vi "Create.vi"(5 "FlexLogger_gRPC in":refnum<class "FlexLogger_gRPC.lvclass">, 8 "error in (no error)":errorcluster, 10 "PortID [Autodetect]":u16, 11 "Address":string="127.0.0.1") -> (0 "error out":errorcluster, 3 "FlexLogger_gRPC out":refnum<class "FlexLogger_gRPC.lvclass">)   [LabVIEW 2020, in "FlexLogger_gRPC.lvlib" / "FlexLogger_gRPC.lvclass"]
doc: "Constructor for the grpc object."
uses:
  FlexLogger_gRPC.lvclass
  FlexLogger_gRPC.lvclass/FlexLogger_gRPC.ctl
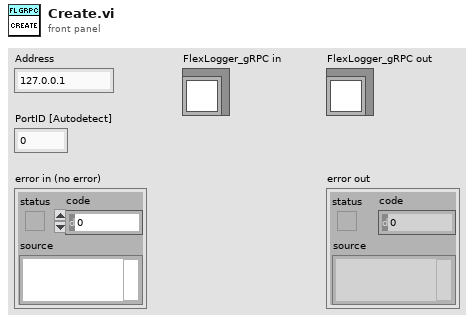
[diagram p1: front panel]
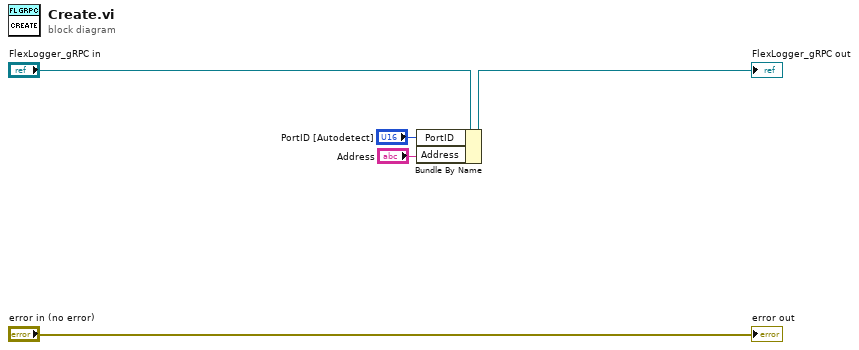
[diagram p0: block diagram]
diagram:
  n1 = Bundle By Name(cluster="FlexLogger_gRPC in", "PortID"="PortID [Autodetect]", "Address"="Address") -> (→"FlexLogger_gRPC out":refnum<class "FlexLogger_gRPC.lvclass">)
  "error out" <- "error in (no error)"
